vi "Add Vectors.vi"(8 "error in":errorcluster, 10 "PVector U":refnum<class "PVector.lvclass">, 11 "PVector V":refnum<class "PVector.lvclass">) -> (0 "error out":errorcluster, 3 "PVector (V+U)":refnum<class "PVector.lvclass">)   [LabVIEW 2016, in "PVector.lvclass"]
doc: "Adds two Vectors by adding their corresponding components. \n<B>V</B>+<B>U</B> == (Vx+Ux, Vy+Uy)"
uses:
  PVector.lvclass
  PVector.lvclass/PVector.ctl
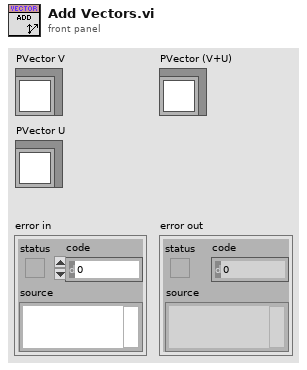
[diagram p1: front panel]
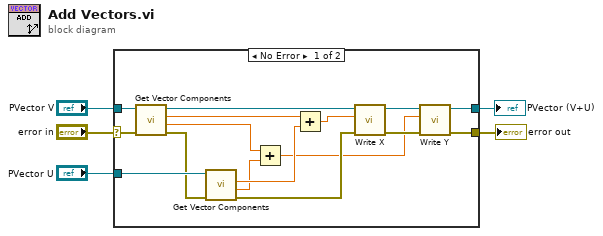
[diagram p0: block diagram]
diagram:
  n1 = case shown="No Error" "error in" {
    selector: "error in" -> [w20 w23]
    tunnel: [w12 w23] -> w4
    tunnel: [w15 w22] -> w2
    tunnel: "PVector V" -> [w21 w22]
    tunnel: "PVector U" -> [w19 _]
    frame No Error {
      n2 = call "Get Vector Components.vi"("error in"=w20, "PVector in"=w21) -> ("error out"=w18:errorcluster, "Y"=w9:dbl, "X"=w11:dbl, "PVector out"=w17:refnum<class "PVector.lvclass">)  [unwired: 6 in]
      n3 = call "Get Vector Components.vi"("error in"=w18, "PVector in"=w19) -> ("error out"=w14:errorcluster, "Y"=w8:dbl, "X"=w10:dbl)  [unwired: 6 in, 1 out]
      n4 = Add(x=w9, y=w8) -> (x+y=w6:dbl)
      n5 = Add(x=w11, y=w10) -> (x+y=w7:dbl)
      n6 = call "Write X.vi"("error in"=w14, "X"=w7, "PVector in"=w17) -> ("error out"=w13:errorcluster, "PVector out"=w16:refnum<class "PVector.lvclass">)  [unwired: 7 in]
      n7 = call "Write Y.vi"("error in"=w13, "Y"=w6, "PVector in"=w16) -> ("error out"=w12:errorcluster, "PVector out"=w15:refnum<class "PVector.lvclass">)  [unwired: 7 in]
    }
    frame Error {
    }
  }
  "error out" <- w4
  "PVector (V+U)" <- w2
